vi "Stop Task.vi"(8 "error in (no error)":errorcluster, 11 "DAQmxTask in":refnum<class "DAQmxTask.lvclass">) -> (0 "error out":errorcluster, 3 "DAQmxTask out":refnum<class "DAQmxTask.lvclass">)   [LabVIEW 2015, in "DAQmxTask.lvclass"]
uses:
  DAQmxTask.lvclass
  DAQmxTask.lvclass/DAQmxTask.ctl
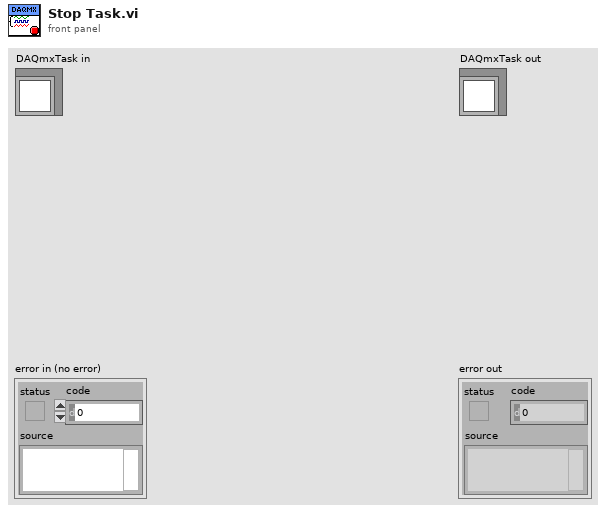
[diagram p1: front panel]
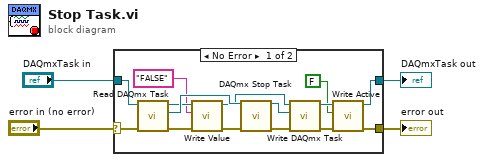
[diagram p0: block diagram]
diagram:
  n1 = case shown="No Error" "error in (no error)" {
    selector: "error in (no error)" -> [w18 w21]
    tunnel: [w13 w21] -> w3
    tunnel: [w14 w20] -> w1
    tunnel: "DAQmxTask in" -> [w19 w20]
    frame No Error {
      n2 = call "Read DAQmx Task.vi"("error in (no error)"=w18, "DAQmxTask in"=w19) -> ("error out"=w10:errorcluster, "DAQmx Task Name"=w8:refnum<k21>, "DAQmxTask out"=w7:refnum<class "DAQmxTask.lvclass">)  [unwired: 7 in]
      n3 = call-dynamic "Write Value.vi"("error in (no error)"=w10, "Data"="FALSE", "DAQmxTask en entrée"=w7) -> ("error out"=w9:errorcluster, "DAQmxTask en sortie"=w5:refnum<class "DAQmxTask.lvclass">)  [unwired: 7 in]
      n4 = call <vilib>:"DAQmx Stop Task.vi"("task/channels in"=w8, "error in"=w9) -> ("task out"=w11:refnum<k21>, "error out"=w12:errorcluster)  [unwired: 12 in]
      n5 = call "Write DAQmx Task.vi"("error in (no error)"=w12, "DAQmx Task Name"=w11, "DAQmxTask in"=w5) -> ("error out"=w17:errorcluster, "DAQmxTask out"=w16:refnum<class "DAQmxTask.lvclass">)  [unwired: 7 in]
      n6 = call-dynamic "Write Active.vi"("error in (no error)"=w17, "Active?"=FALSE, "DAQmxTask in"=w16) -> ("error out"=w13:errorcluster, "DAQmxTask out"=w14:refnum<class "DAQmxTask.lvclass">)  [unwired: 7 in]
    }
    frame Error {
    }
  }
  "error out" <- w3
  "DAQmxTask out" <- w1
